vi "sub_GSlam_cal-edges.vi"(10 "z_list":dbl[][][](array[numeric]), 11 "x_list":cluster{"x":dbl, "y":dbl, "yaw":dbl}[](array[cluster])) -> (2 "cost":dbl, 3 "edge arr":T2(array[cluster]))   [LabVIEW 2019]
uses:
  <vilib>/Analysis/Matrix/Datatypes/RealMatrix.ctl
  Ctrl/cmd_ini-add-read.ctl
  Ctrl/cmd_common.ctl
  Ctrl/cmd_ini-RW.ctl
  <vilib>/Analysis/Matrix/Numeric/Multiply/Multiply - RM,RM.vi
  <vilib>/Analysis/Matrix/NI_Matrix.lvlib
panel:
  out "cnt":u32
  out "cost":dbl(graph)
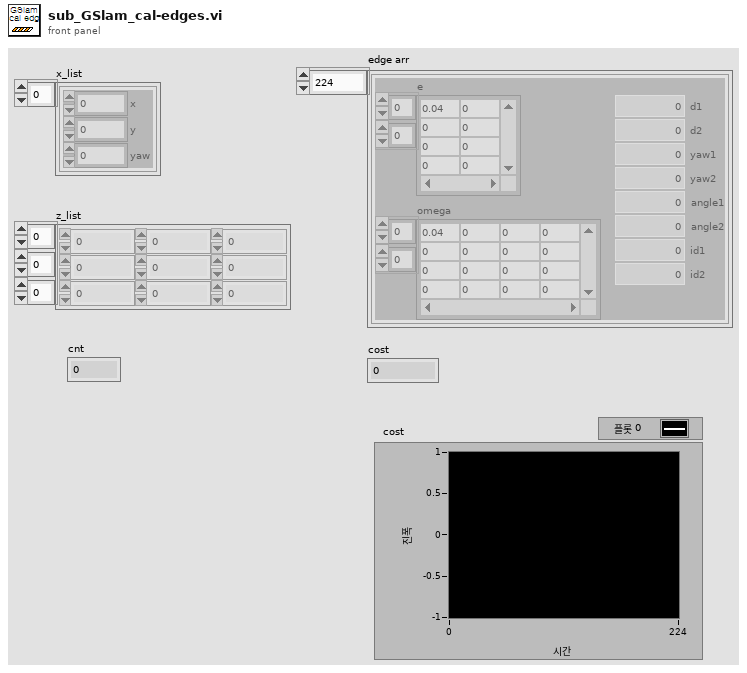
[diagram p1: front panel]
types:
  T1 = typedef "NI_Matrix.lvlib/RealMatrix.ctl" = dbl[][]
  T2 = cluster{"e":T1, "omega":T1, "d1":dbl, "d2":dbl, "yaw1":dbl, "yaw2":dbl, "angle1":dbl, "angle2":dbl, "id1":i32, "id2":i32}[]
  T3 = typedef "cmd_ini-add-read.ctl" = enum16{"ini", "add", "read"}
  T4 = cluster{"x_dr":cluster{"x":dbl, "y":dbl, "yaw":dbl}, "x_dr":cluster{"x":dbl, "y":dbl, "yaw":dbl}, "d1":dbl, "angle1":dbl, "d2":dbl, "angle2":dbl, "t1":i32, "t2":i32}
  T5 = typedef "cmd_ini-RW.ctl" = enum16{"ini", "read", "write"}
  T6 = typedef "cmd_common.ctl" = enum16{"read", "write"}
  T7 = typedef "slam_edge.ctl" = cluster{"e":T1, "omega":T1, "d1":dbl, "d2":dbl, "yaw1":dbl, "yaw2":dbl, "angle1":dbl, "angle2":dbl, "id1":i32, "id2":i32}
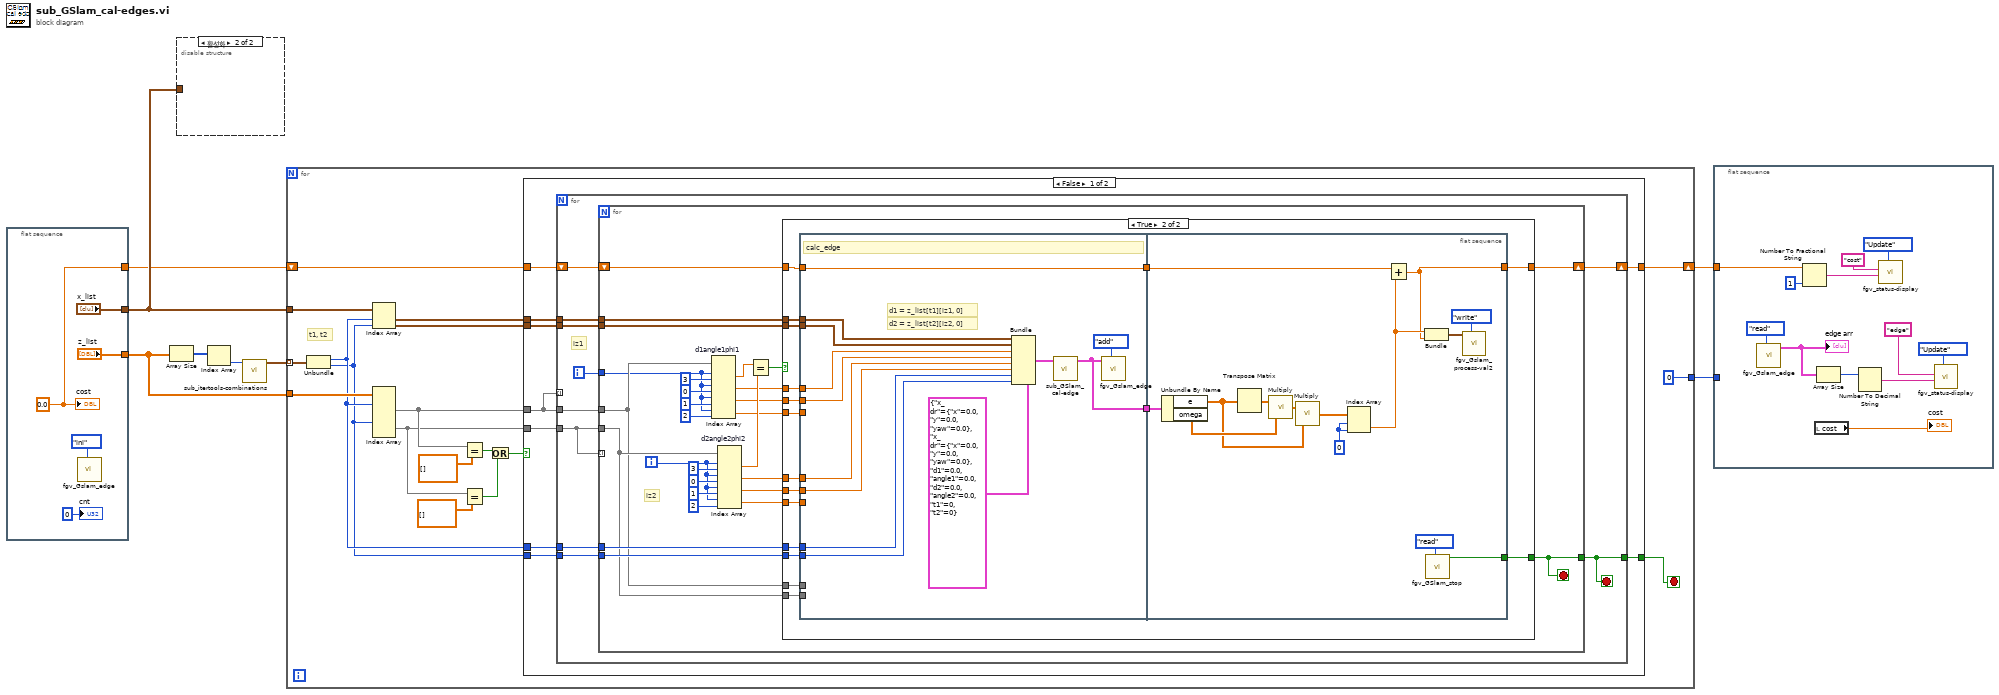
[diagram p0: block diagram]
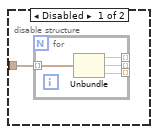
[diagram p2: hidden frame]
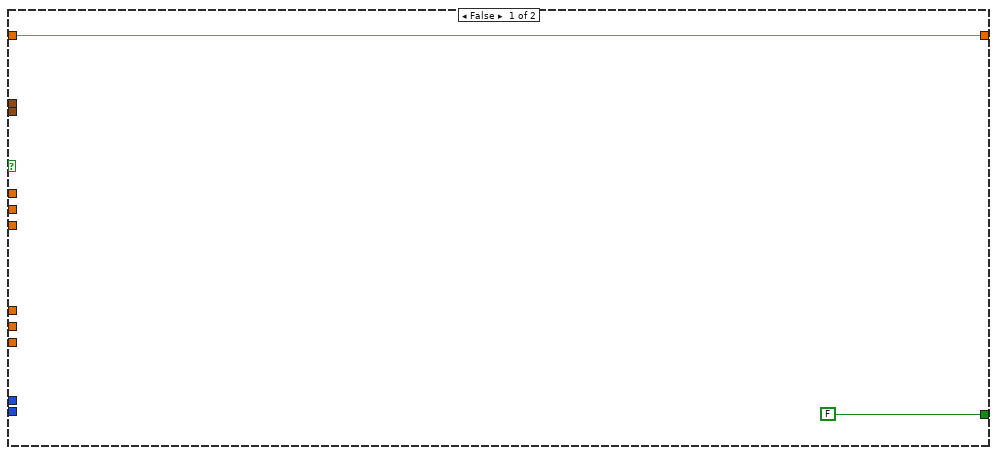
[diagram p3: hidden frame]
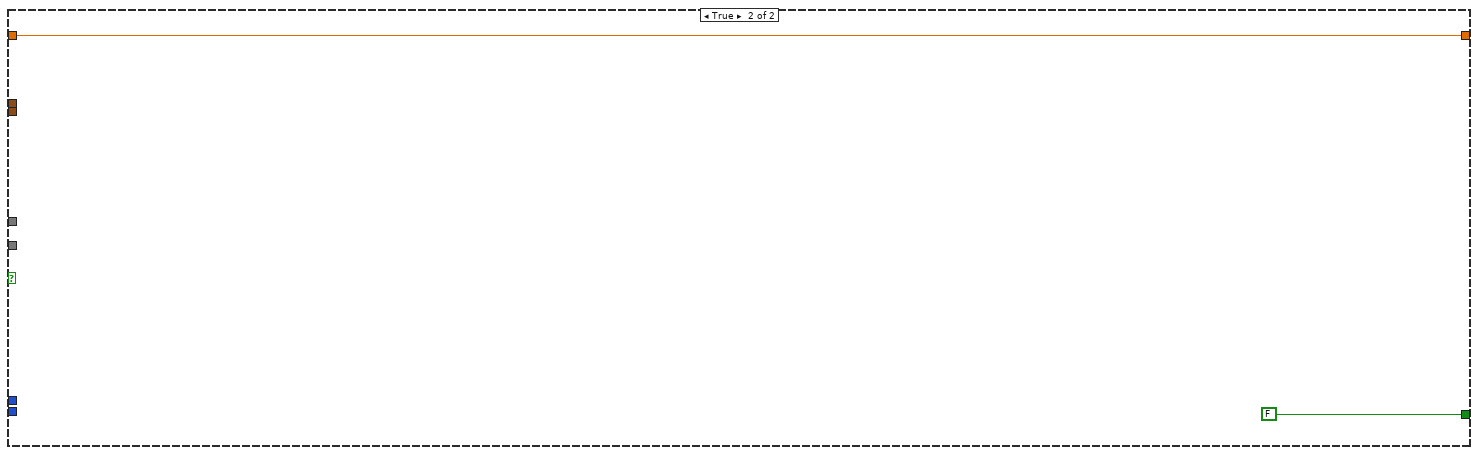
[diagram p4: hidden frame]
diagram:
  n1 = flat-sequence {
    tunnel: ["x_list"] -> w5
    tunnel: ["z_list"] -> w4
    tunnel: [w10] -> w2
    frame #0 {
      w10 = 0.0 ("cost")
      n2 = call "fgv_Gslam_edge.vi"("cmd"=cmd_ini-add-read."ini") -> ()  [unwired: 10 in, 1 out]
      "cost" <- w10
      "cnt" <- u32 0 ("cnt")
    }
  }
  n3 = Array Size(array=w4) -> (size(s)=w8:i32[])
  n4 = disable-structure shown="활성화" {
    disable-tunnel: w5 -> [w14 _]
    frame Disabled {
      n5 = for {
        tunnel: w14 -> [w18] mode=indexing
        tunnel: [w17] -> _ mode=indexing
        tunnel: [w16] -> _ mode=indexing
        tunnel: [w15] -> _ mode=indexing
        n6 = Unbundle(w18) -> ("x"=w17:dbl, "y"=w16:dbl, "yaw"=w15:dbl)
      }
    }
    frame Enabled {
    }
  }
  n7 = Index Array(array=w8) -> (element=w7:i32)  [unwired: 1 in]
  n8 = call "sub_itertools-combinations.vi"("N"=w7) -> ("z_ids"=w6:cluster{"x":i32, "y":i32}[])  [unwired: 10 in]
  n9 = for {
    tunnel: w6 -> [w36] mode=indexing
    tunnel: w5 -> [w35]
    tunnel: w4 -> [w29]
    tunnel: [0] -> w3
    shift-right: [w20] -> w1
    shift-left: w2 -> [w21]
    stop <- w19 stop-if-true
    # "t1, t2"
    n10 = Unbundle(w36) -> ("x"=w24:i32, "y"=w23:i32)
    n11 = Index Array(array=w35, index #1=w24, index #2=w23) -> (element #1=w26:cluster{"x":dbl, "y":dbl, "yaw":dbl}, element #2=w25:cluster{"x":dbl, "y":dbl, "yaw":dbl})
    n12 = Index Array(array=w29, index (dim 0) #1=w24, index (dim 0) #2=w23) -> (element #1=w28:dbl[][], element #2=w27:dbl[][])  [unwired: 4 in]
    n13 = Equal?(x=w28, y=dbl[][] []) -> (x = y?=w30:bool)
    n14 = Equal?(x=w27, y=dbl[][] []) -> (x = y?=w31:bool)
    n15 = Or(x=w30, y=w31) -> (x .or. y?=w32:bool)
    n16 = case shown="False" w32 {
      tunnel: w28 -> [w44 _]
      tunnel: w27 -> [w45 _]
      tunnel: w26 -> [w43 _]
      tunnel: w25 -> [w42 _]
      tunnel: w24 -> [w41 _]
      tunnel: w23 -> [w40 _]
      tunnel: w21 -> [w39 w131]
      tunnel: [w38 w131] -> w20
      tunnel: [w37 FALSE ("val")] -> w19
      frame False {
        n17 = for {
          tunnel: w44 -> [w55]
          tunnel: w45 -> [w53]
          tunnel: w44 -> [_] mode=indexing
          tunnel: w43 -> [w52]
          tunnel: w42 -> [w51]
          tunnel: w41 -> [w50]
          tunnel: w40 -> [w49]
          shift-right: [w47] -> w38
          shift-left: w39 -> [w48]
          tunnel: [w46] -> w37
          i -> [w54]
          stop <- w46 stop-if-true
          # "iz1"
          n18 = for {
            tunnel: w55 -> [w61]
            tunnel: w53 -> [w62]
            tunnel: w54 -> [w60]
            tunnel: w53 -> [_] mode=indexing
            tunnel: w52 -> [w66]
            tunnel: w51 -> [w65]
            tunnel: w50 -> [w64]
            tunnel: w49 -> [w63]
            shift-right: [w57] -> w47
            shift-left: w48 -> [w58]
            tunnel: [w56] -> w46
            i -> [w59]
            stop <- w56 stop-if-true
            # "iz2"
            n19 = Index Array "d1angle1phi1"(array=w61, index (row) #1=w60, index (col) #1=3 ("disabled index (col)"), index (row) #2=w60, index (col) #2=0 ("disabled index (col)"), index (row) #3=w60, index (col) #3=1 ("disabled index (col)"), index (row) #4=w60, index (col) #4=2 ("disabled index (col)")) -> (element #1=w80:dbl, element #2=w77:dbl, element #3=w73:dbl, element #4=w69:dbl)
            n20 = Index Array "d2angle2phi2"(array=w62, index (row) #1=w59, index (col) #1=3 ("disabled index (col)"), index (row) #2=w59, index (col) #2=0 ("disabled index (col)"), index (row) #3=w59, index (col) #3=1 ("disabled index (col)"), index (row) #4=w59, index (col) #4=2 ("disabled index (col)")) -> (element #1=w81:dbl, element #2=w75:dbl, element #3=w71:dbl, element #4=w67:dbl)
            n21 = Equal?(x=w80, y=w81) -> (x = y?=w79:bool)
            n22 = case shown="True" w79 {
              tunnel: w77 -> [_ w102]
              tunnel: w75 -> [_ w99]
              tunnel: w73 -> [_ w101]
              tunnel: w71 -> [_ w98]
              tunnel: w69 -> [_ w100]
              tunnel: w67 -> [_ w97]
              tunnel: w66 -> [_ w96]
              tunnel: w65 -> [_ w95]
              tunnel: w64 -> [_ w94]
              tunnel: w63 -> [_ w93]
              tunnel: w62 -> [_ w91]
              tunnel: w61 -> [_ w90]
              tunnel: w58 -> [w85 w89]
              tunnel: [w85 w87] -> w57
              tunnel: [FALSE ("val") w86] -> w56
              frame False {
              }
              frame True {
                n23 = flat-sequence {
                  tunnel: w102 -> [w113]
                  tunnel: w101 -> [w112]
                  tunnel: w100 -> [_]
                  tunnel: w99 -> [w110]
                  tunnel: w98 -> [w111]
                  tunnel: w97 -> [_]
                  tunnel: w96 -> [w115]
                  tunnel: w95 -> [w114]
                  tunnel: w94 -> [w107]
                  tunnel: w93 -> [w106]
                  tunnel: [w108] -> w92
                  tunnel: w91 -> [_]
                  tunnel: w90 -> [_]
                  tunnel: w89 -> [w103]
                  tunnel: [w103] -> w88
                  tunnel: w92 -> [w129]
                  tunnel: w88 -> [w122]
                  tunnel: [w119] -> w87
                  tunnel: [w116] -> w86
                  frame #0 {
                    # "d2 = z_list[t2][iz2, 0]"
                    # "d1 = z_list[t1][iz1, 0]"
                    # "calc_edge"
                    n24 = Bundle(cluster=T4 {"x_dr"={"x"=0.0, "y"=0.0, "yaw"=0.0}, "x_dr"={"x"=0.0, "y"=0.0, "yaw"=0.0}, "d1"=0.0, "angle1"=0.0, "d2"=0.0, "angle2"=0.0, "t1"=0, "t2"=0}, "x_dr"=w115, "x_dr"=w114, "d1"=w113, "angle1"=w112, "d2"=w110, "angle2"=w111, "t1"=w107, "t2"=w106) -> (w105:T4)
                    n25 = call "sub_GSlam_cal-edge.vi"("in"=w105) -> ("edge out"=w108:T7)  [unwired: 10 in]
                    n26 = call "fgv_Gslam_edge.vi"("cmd"=cmd_ini-add-read."add", "edge"=w108) -> ()  [unwired: 9 in, 1 out]
                  }
                  frame #1 {
                    w123 = 0 ("인덱스 (행)")
                    n27 = Unbundle By Name(w129) -> ("e"=w125:T1, "omega"=w127:T1)
                    n28 = Transpose Matrix(1:w125) -> (0:w128:T1)
                    n29 = call-poly <vilib>:"Multiply.vi"("Real Matrix B"=w127, "Real Matrix A"=w128) -> ("A * B"=w126:T1)
                    n30 = call-poly <vilib>:"Multiply.vi"("Real Matrix B"=w125, "Real Matrix A"=w126) -> ("A * B"=w124:T1)
                    n31 = Index Array(array=w124, index (row)=w123, index (col)=w123) -> (element=w120:dbl)
                    n32 = Add(x=w122, y=w120) -> (x+y=w119:dbl)
                    n33 = Bundle("Real Matrix Element"=w120, w119) -> (w118:cluster{"Real Matrix Element":dbl, dbl})  [unwired: 1 in]
                    n34 = call "fgv_GSlam_stop.vi"("cmd"=cmd_ini-RW."read") -> ("val"=w116:bool)  [unwired: 10 in]
                    n35 = call "fgv_Gslam_process-val2.vi"("cmd"=cmd_common."write", "data"=w118) -> ()  [unwired: 9 in, 1 out]
                  }
                }
              }
            }
          }
        }
      }
      frame True {
      }
    }
  }
  n36 = flat-sequence {
    tunnel: w3 -> [_]
    tunnel: w1 -> [w132]
    frame #0 {
      n37 = call "fgv_Gslam_edge.vi"("cmd"=cmd_ini-add-read."read") -> ("edge arr"=w142:T2)  [unwired: 10 in]
      "edge arr" <- w142
      n38 = Number To Fractional String(number=w132, precision (6)=i16 1 ("정밀도(6)")) -> (F-format string=w136:string)  [unwired: 2 in]
      n39 = local read "cost"() -> (→"cost":dbl)
      n40 = Array Size(array=w142) -> (size(s)=w138:i32)
      n41 = Number To Decimal String(number=w138) -> (decimal integer string=w139:string)  [unwired: 1 in]
      n42 = call "fgv_status-display.vi"("Mode"=enum16{"Initial", "Update", "Clear"}."Update", "detail"=w136, "title"="cost") -> ()  [unwired: 8 in, 1 out]
      n43 = call "fgv_status-display.vi"("Mode"=enum16{"Initial", "Update", "Clear"}."Update", "detail"=w139, "title"="edge") -> ()  [unwired: 8 in, 1 out]
    }
  }
